vi "make_key.vi"(11 "gonghao":string) -> (2 "key_out":string)   [LabVIEW 2017, in "Lib_code.lvlib"]
uses:
  Lib_code.lvlib
panel:
  out "64位整型":i64
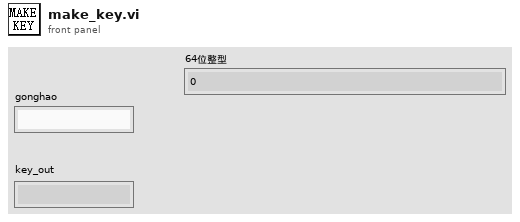
[diagram p1: front panel]
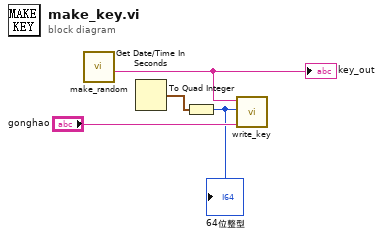
[diagram p0: block diagram]
diagram:
  n1 = call "make_random.vi"() -> ("key"=w4:string)  [unwired: 11 in]
  "key_out" <- w4
  n2 = Get Date/Time In Seconds() -> (seconds since 1Jan1904=w2:timestamp)
  n3 = To Quad Integer(1:w2) -> (0:w1:i64)
  "64位整型" <- w1
  n4 = call "write_key.vi"("file_name"="gonghao", "time"=w1, "key"=w4) -> ()  [unwired: 9 in]
